vi "Measurement UI.vi"() -> ()   [LabVIEW 2021, in "Efficiency Sweep_Class D Amplifier_UI.lvlib"]
uses:
  Efficiency Sweep_Class D Amplifier_UI.lvlib
  shared/controls/units - snr.ctl
  shared/controls/units - ratio.ctl
  shared/controls/digital output level units.ctl
  shared/ui/controls/view.ctl
  shared/controls/power measurement method.ctl
  UI State.ctl
  <vilib>/Utility/miscctls.llb/LVBoundsTypeDef.ctl
  <vilib>/Utility/miscctls.llb/LVPoint32TypeDef.ctl
  <vilib>/Utility/miscctls.llb/LVPointTypeDef.ctl
  shared/ui/UI Helpers.lvlib
  shared/audio popup ui/Audio Popup UI.lvlib
  shared/controls/audio controls.lvlib
panel:
  in  "view legend":T1
  out "plot point":string
  out "Sweep graph":cluster{"frequency (Hz)":dbl[], "THD+N":dbl[]}[](graph)
  out "Time domain graph":waveform(dbl)(graph)
  out "Frequency domain graph":T2(graph)
  in  "digital serial cfg file":string
  in  "power measurement resource":string="PXI1Slot4/ai0"
  out "efficiency (%)":dbl[](array[numeric])
  out "power loss (W)":dbl[](array[numeric])
  out "total output power (W)":dbl[](array[numeric])
  out "input power (W)":dbl[](array[numeric])
  out "power supply current (A)":dbl[](array[numeric])
  out "power supply voltage (V)":dbl[](array[numeric])
  in  "Configuration tab":enum32{"Protocol", "Measurement", "Units"}(tab)
  out "digital serial file name":string
  in  "configure digital serial":bool
  in  "master clock channel list":string caption="Master Clock Channel"
  in  "digital channel list":string caption="Digital Audio Channel"
  in  "output level units 2":T3
  in  "sense resistor (Ohms)":dbl caption="Sense Resistor" format="%#_g Ohms"
  in  "power supply current limit":dbl caption="Current Limit" format="%#_g A"
  in  "power supply voltage":dbl caption="Power Supply Voltage" format="%#_g V"
  in  "power meas resource":refnum<k15> caption="Resource"
  in  "power measurement method":T4 caption="Method"
  in  "output level units":T3
  in  "min settling cycles":u32 caption="Minimum settling cycles"
  in  "min settling time (s)":dbl=0.1 caption="Minimum settling time" format="%#_6ps"
  in  "output sweep number of steps":u32=20000 caption="Number of steps"
  in  "output level start":dbl=20.0 caption="Sweep start" format="%#_6p"
  in  "output level stop":dbl=20000.0 caption="Sweep stop"
  in  "min measurement cycles":u32 caption="Minimum measurement cycles"
  in  "Acquisition channel":tag
  in  "acq sampling rate":dbl=51200.0 caption="Sample rate" format="%#.6pHz"
  in  "min measurement time (s)":dbl=0.1 caption="Minimum measurement time" format="%#_6ps"
  in  "lowpass filter":T5(ring) caption="Lowpass filter"
  in  "highpass filter":enum32{"DC", "AC"}(ring) caption="Highpass filter"
  in  "band start":dbl=20.0 caption="Band start" format="%#_6pHz"
  in  "band stop":dbl=20000.0 caption="Band stop" format="%#_6pHz"
  in  "weighting filter":T6(ring)=enum."A-weighting" caption="Weighting filter"
  in  "load impedance":dbl=4.0 caption="Load impedance" format="%#_6p Ohms"
  in  "output range (pk-pk)":dbl=15.0 caption="Output range" format="%.3p Vpk-pk"
  in  "gain units":T7 caption="Gain"
  in  "THD units":T7 caption="THD"
  in  "THD+N units":T7 caption="THD+N"
  in  "SNR units":T8 caption="SNR"
  in  "channel 0 offset":u32=1
  out "fft - data":dbl[](array[numeric])
  out "fft - df":dbl
  out "fft - f0":dbl
  out "wfm - data":dbl[](array[numeric])
  out "wfm - dt":dbl
  out "wfm - t0":dbl
  out "channel name":string
  in  "acq channel":string="PXI1Slot4/ai0"
  in  "signal phase":dbl caption="phase"
  # "hidden controls - used to sync with MeasLink"
  # "hidden indicators"
  # "Digital Serial Settings"
  # "Harware Resource"
  # "Output Sweep"
  # "Filters"
  # "Acquisition"
  # "Power"
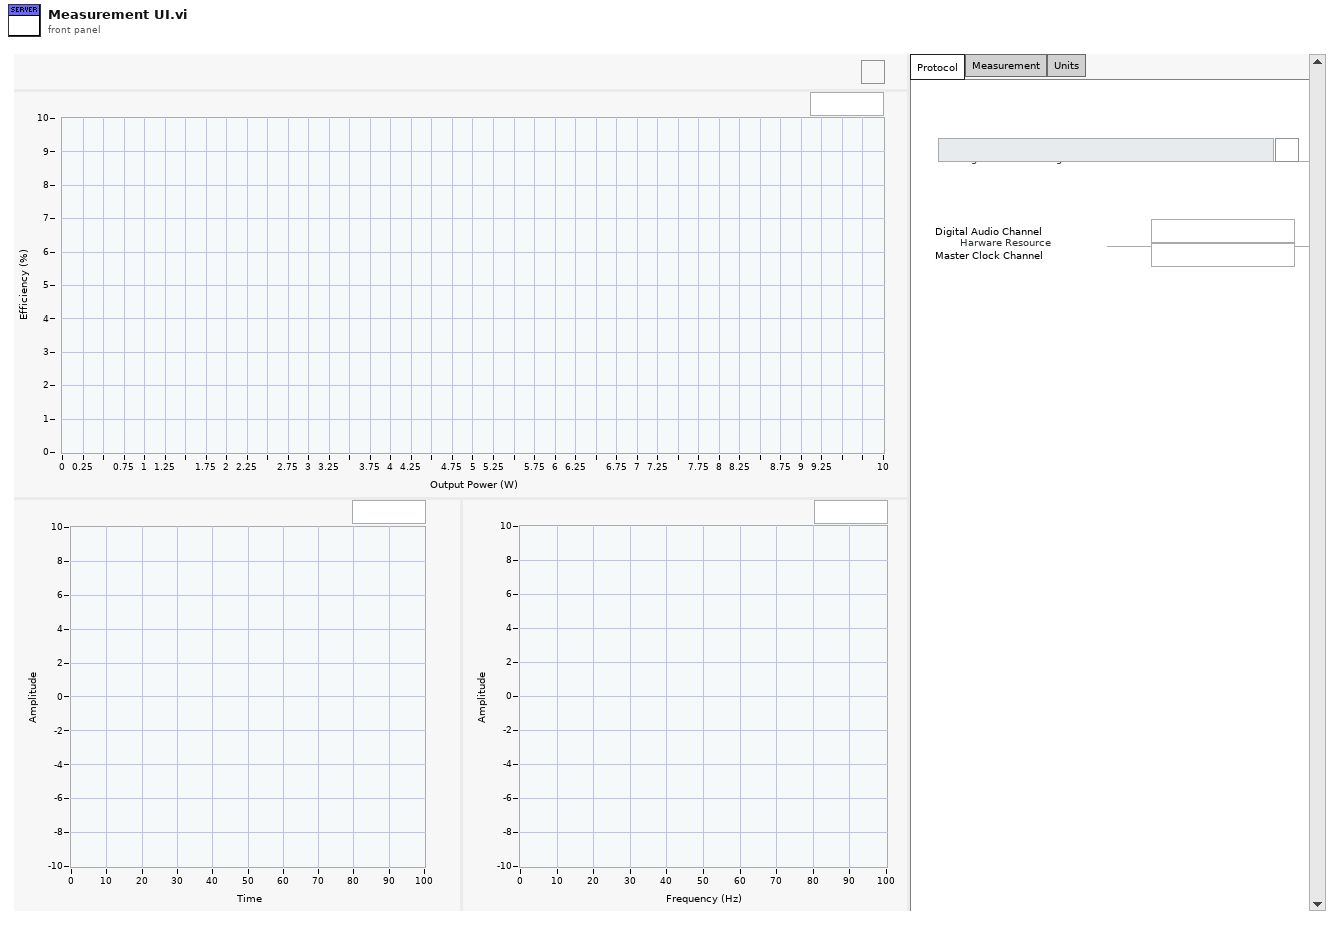
[diagram p1: front panel]
types:
  T1 = typedef "UI Helpers.lvlib/view.ctl" = bool
  T2 = cluster{"fft - f0":dbl, "fft - df":dbl, "fft - data":dbl[]}
  T3 = typedef "audio controls.lvlib/digital output level units.ctl" = enum32{"% FS", "dBFS", "V"}
  T4 = typedef "power measurement method.ctl" = enum32{"SMU", "DMM"}
  T5 = enum32{"No filter", "AES17 20kHz", "AES17 40kHz"}
  T6 = enum32{"Linear", "A-weighting", "B-weighting", "C-weighting"}
  T7 = typedef "audio controls.lvlib/units - ratio.ctl" = enum32{"dB", "%", "x/y"}
  T8 = typedef "audio controls.lvlib/units - snr.ctl" = enum32{"dB", "x/y"}
  T9 = typedef "Efficiency Sweep_Class D Amplifier_UI.lvlib/UI State.ctl" = cluster{"Graph Size":T10, "Legend Visible":bool, "Mouse Coords":T11, "Visible Plot Id":i32, "PostUI event occurred":bool, "digital serial cfg file":path}
  T10 = typedef "LVBoundsTypeDef.ctl" = cluster{"Width":u32, "Height":u32}
  T11 = typedef "LVPoint32TypeDef.ctl" = cluster{"Horizontal":i32, "Vertical":i32}
  T12 = typedef "LVPointTypeDef.ctl" = cluster{"Horizontal":i16, "Vertical":i16}
  T13 = typedef "Audio Popup UI.lvlib/audio settings.ctl" = cluster{"digital serial file":string}
  T14 = cluster{"total output power (W)":dbl[], "efficiency (%)":dbl[]}
  T15 = cluster{"total output power (W)":dbl[], "power loss (W)":dbl[]}
  T16 = cluster{"total output power (W)":dbl[], "input power (W)":dbl[]}
  T17 = cluster{"total output power (W)":dbl[], "input power (W)":dbl[]}[]
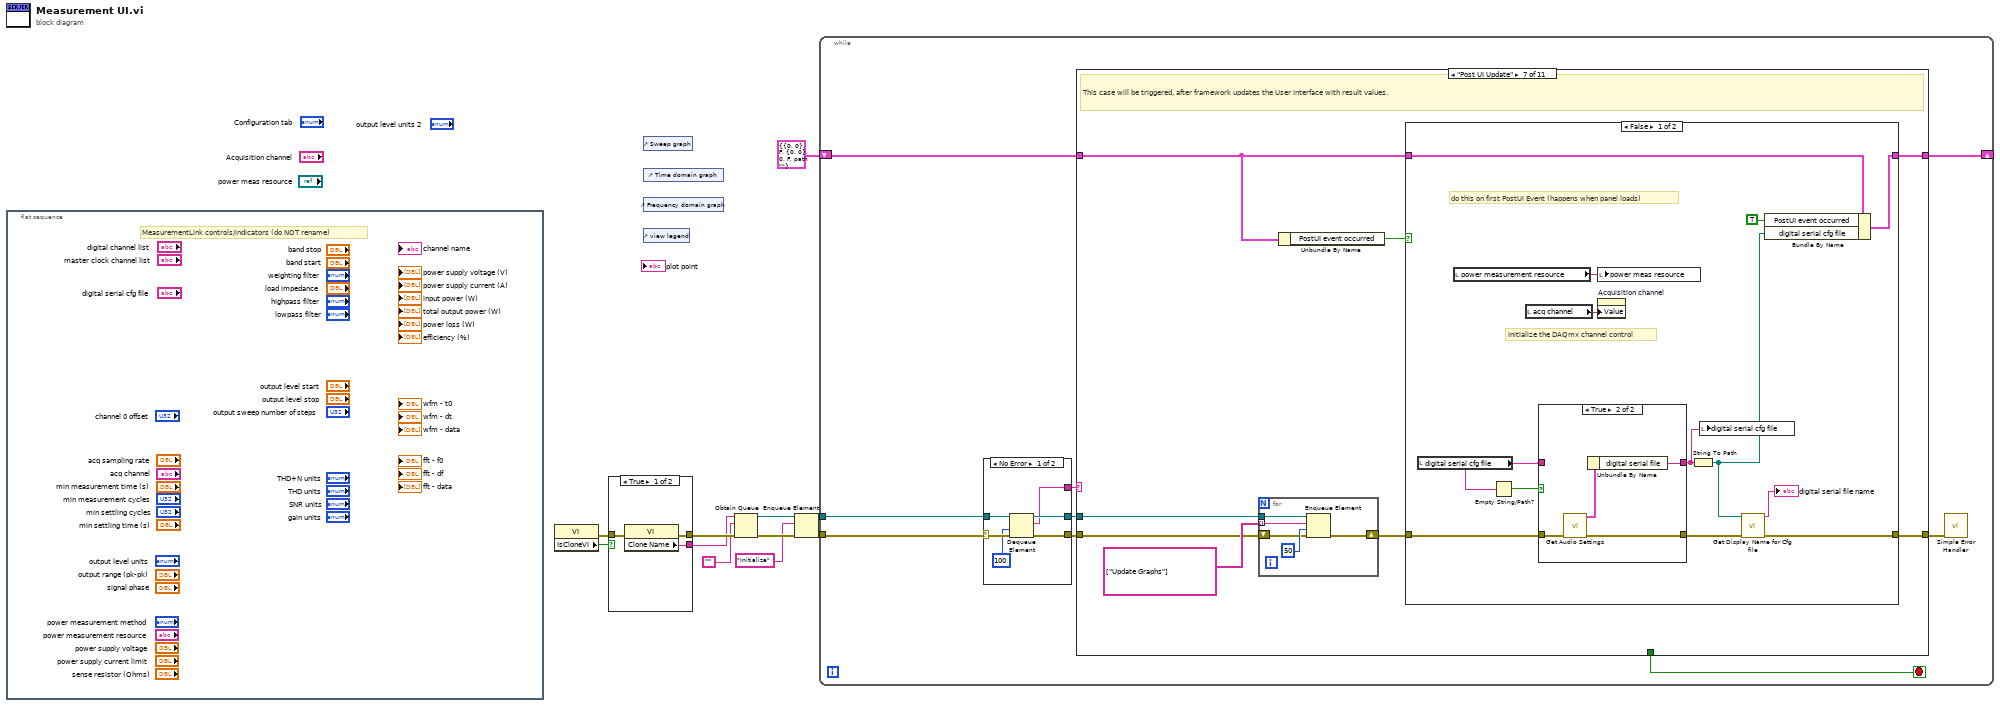
[diagram p0: block diagram]
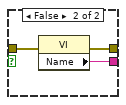
[diagram p2: hidden frame]
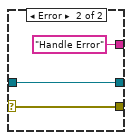
[diagram p3: hidden frame]
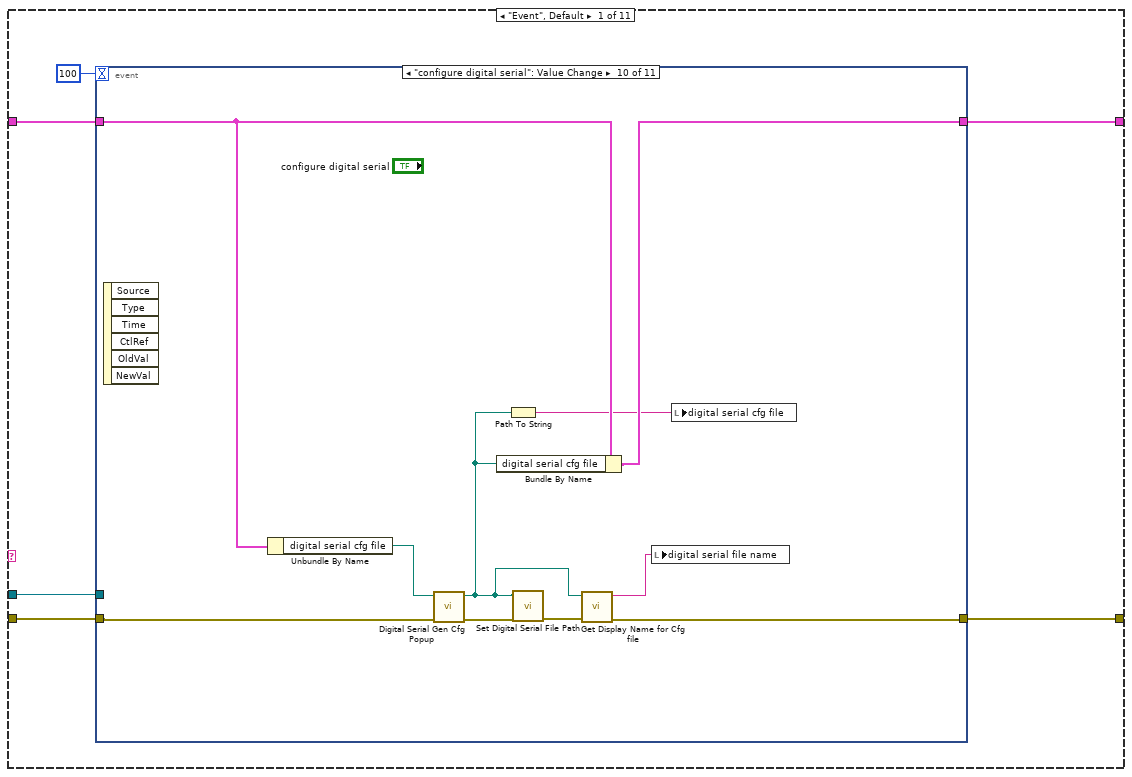
[diagram p4: hidden frame]
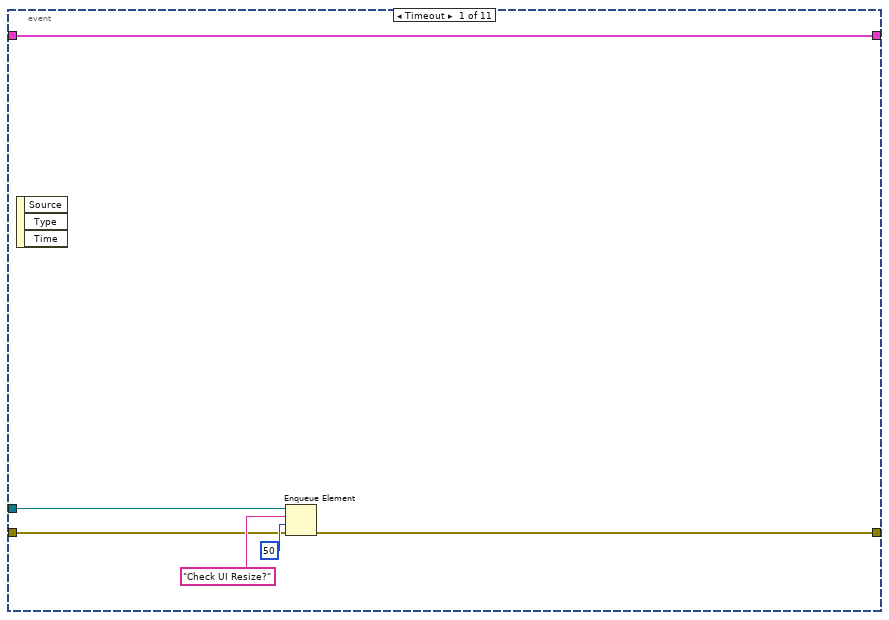
[diagram p5: hidden frame]
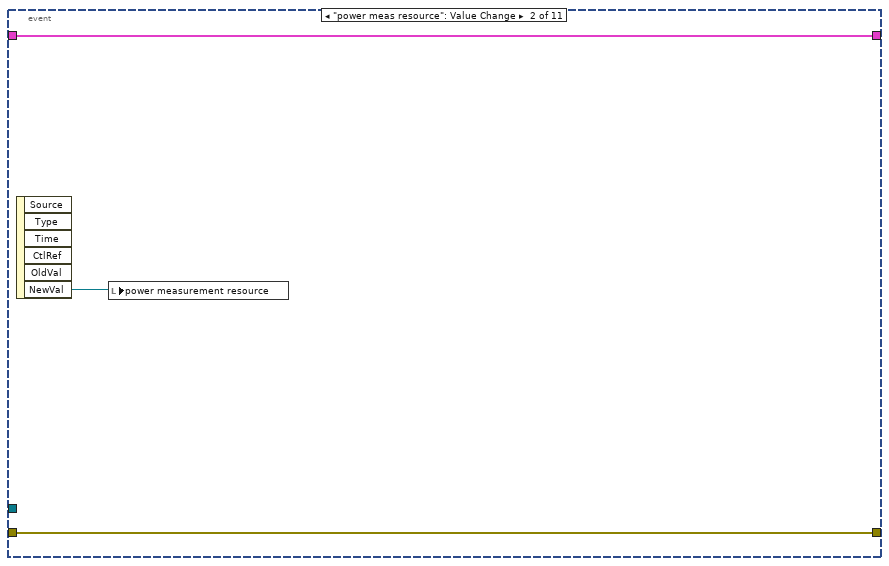
[diagram p6: hidden frame]
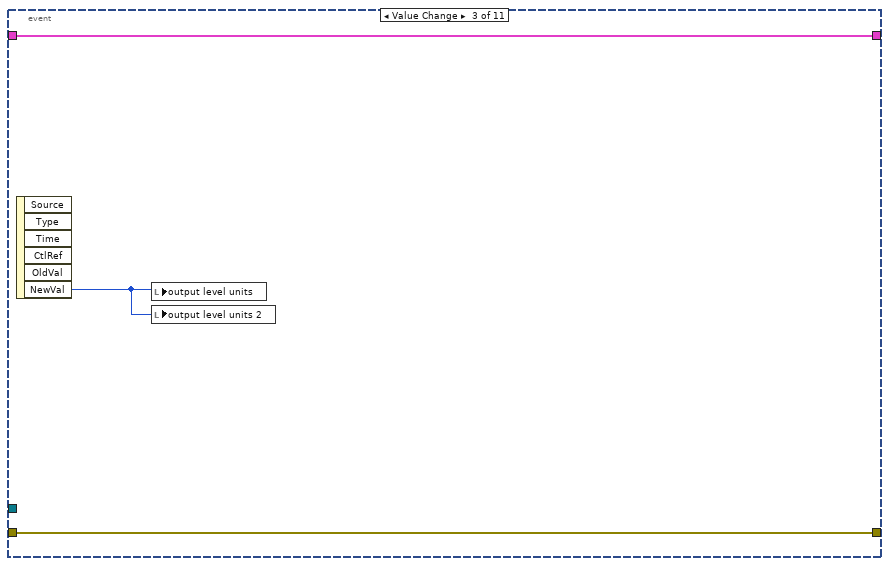
[diagram p7: hidden frame]
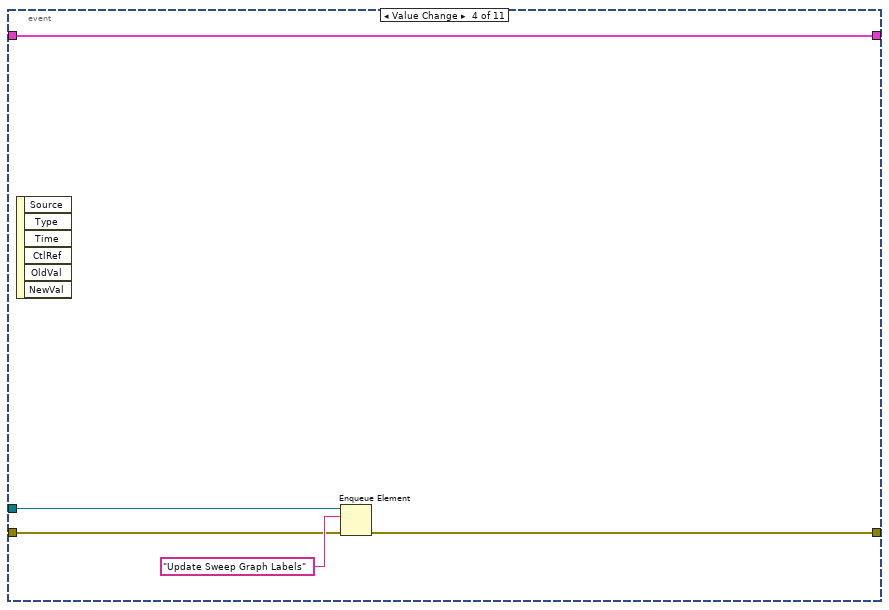
[diagram p8: hidden frame]
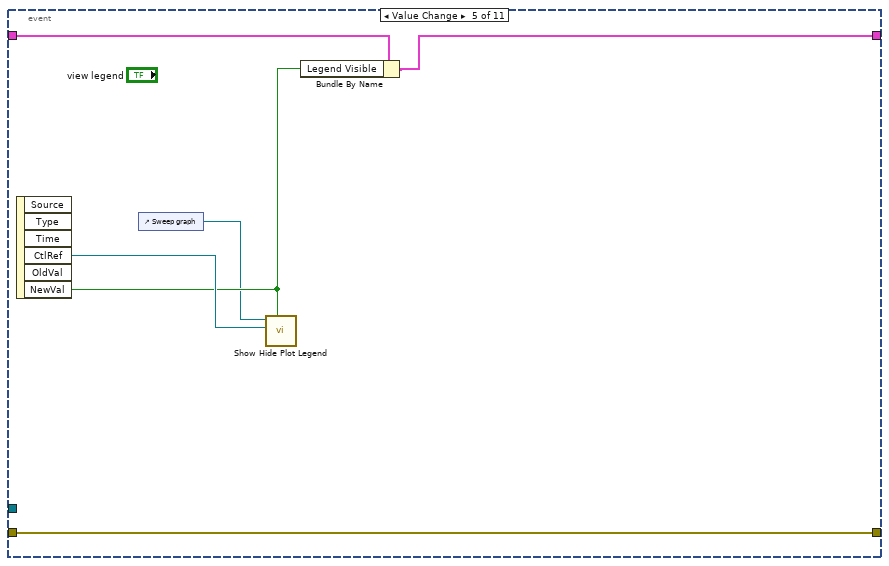
[diagram p9: hidden frame]
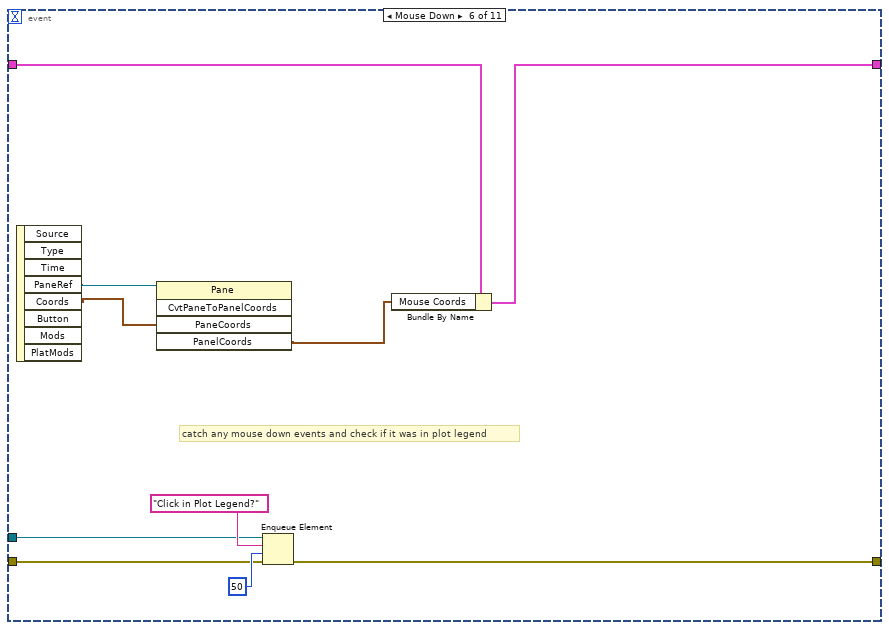
[diagram p10: hidden frame]
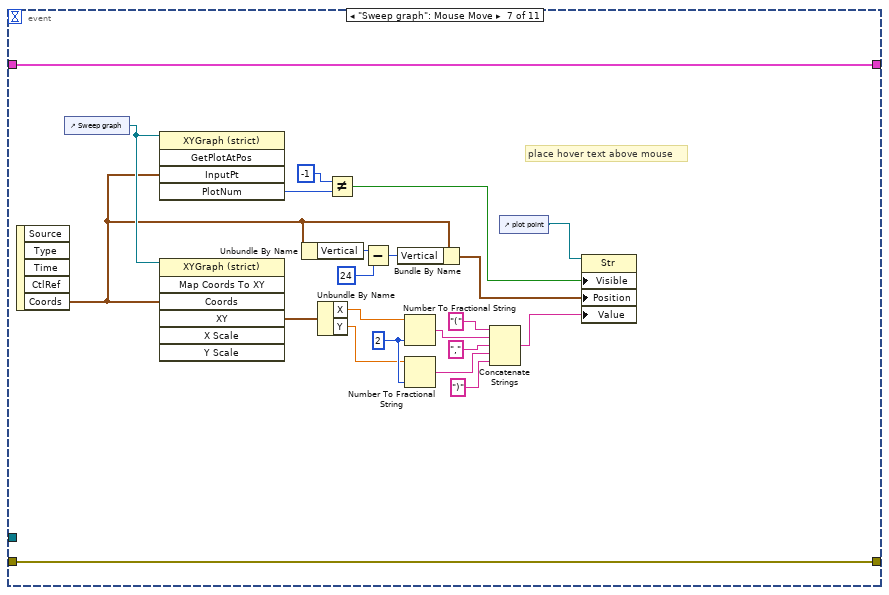
[diagram p11: hidden frame]
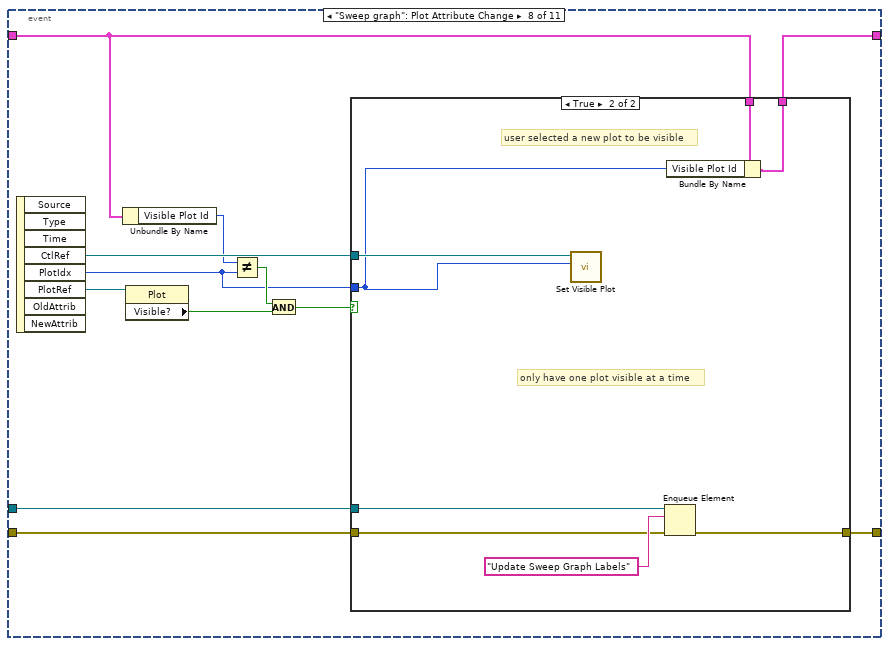
[diagram p12: hidden frame]
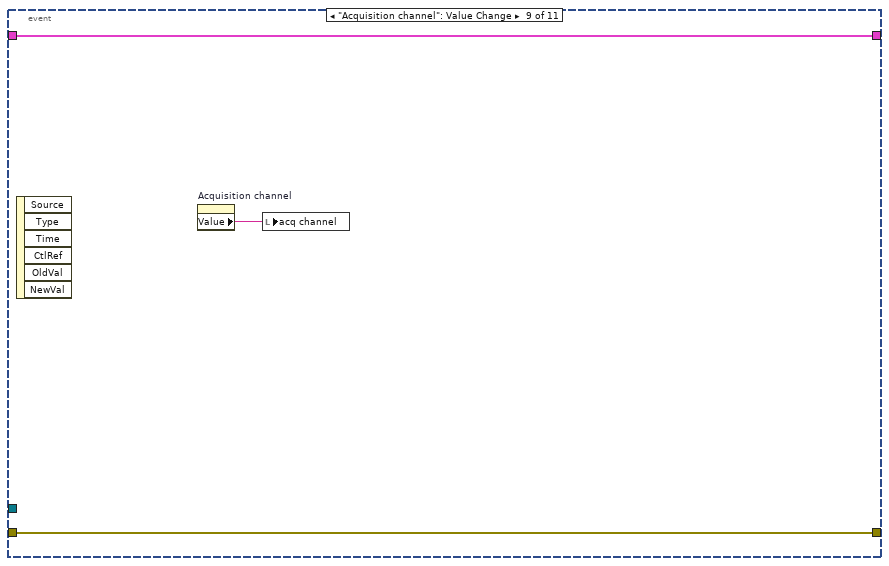
[diagram p14: hidden frame]
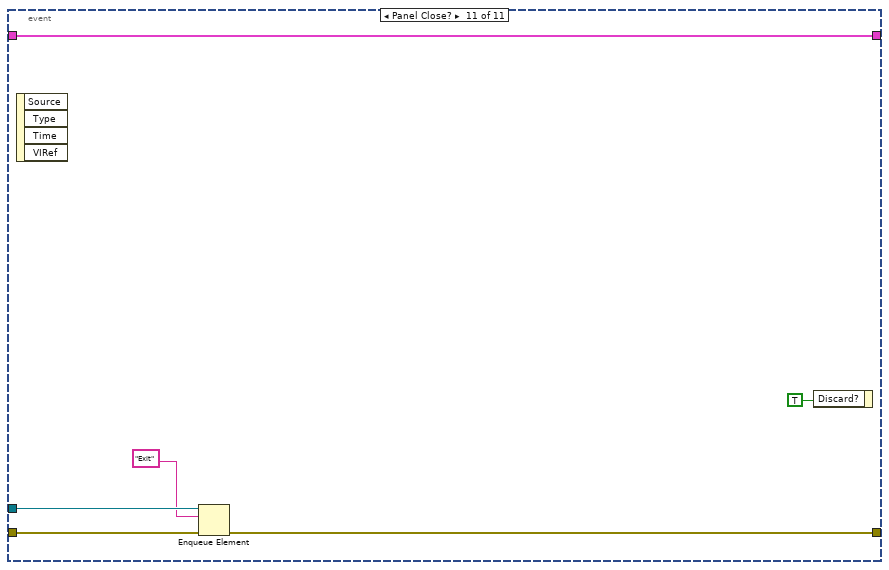
[diagram p15: hidden frame]
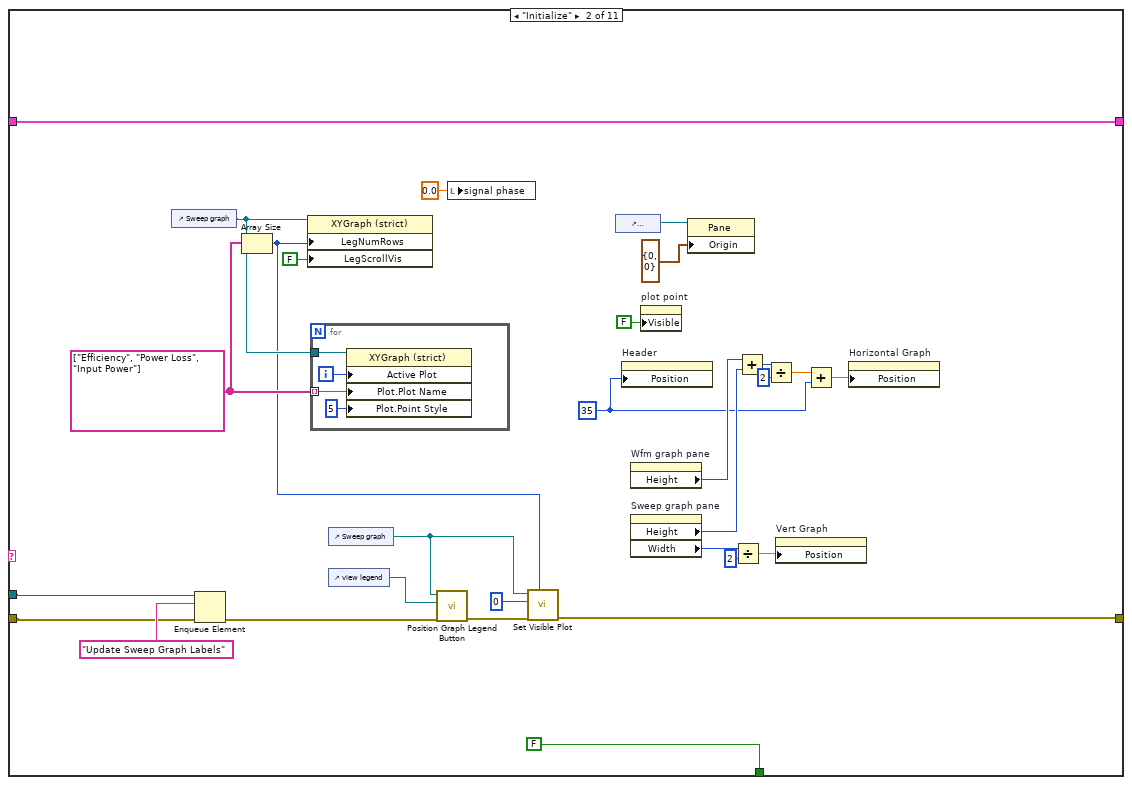
[diagram p16: hidden frame]
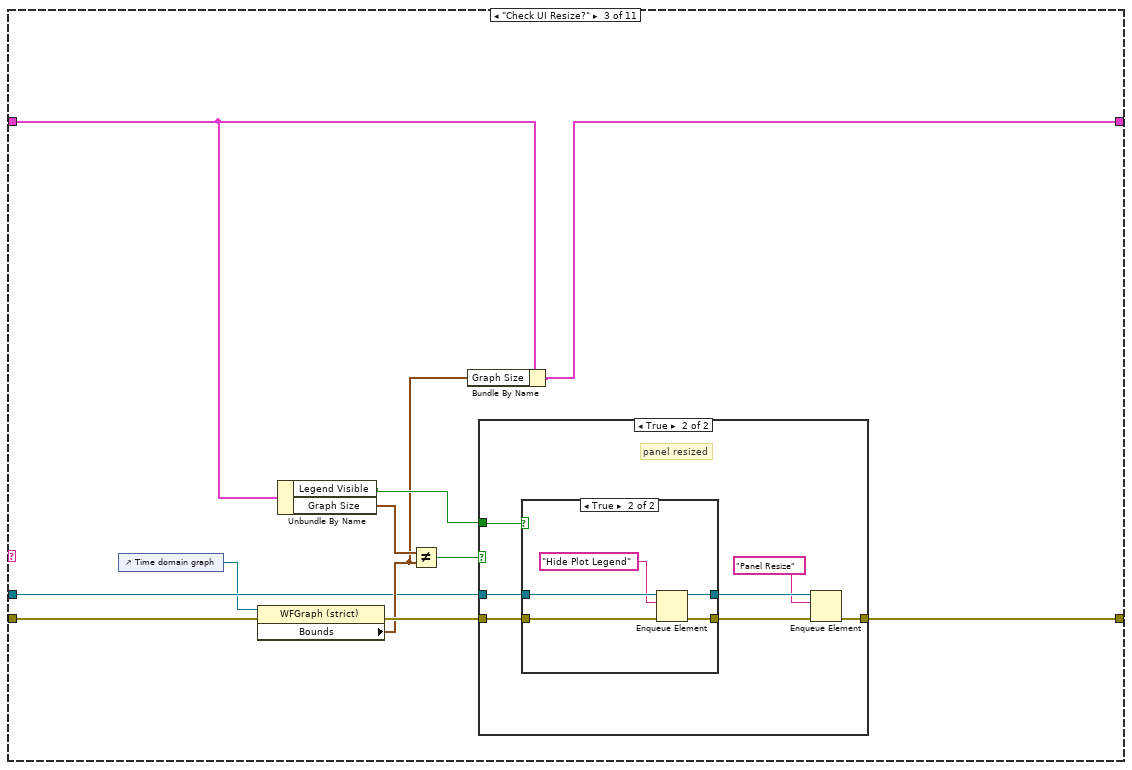
[diagram p17: hidden frame]
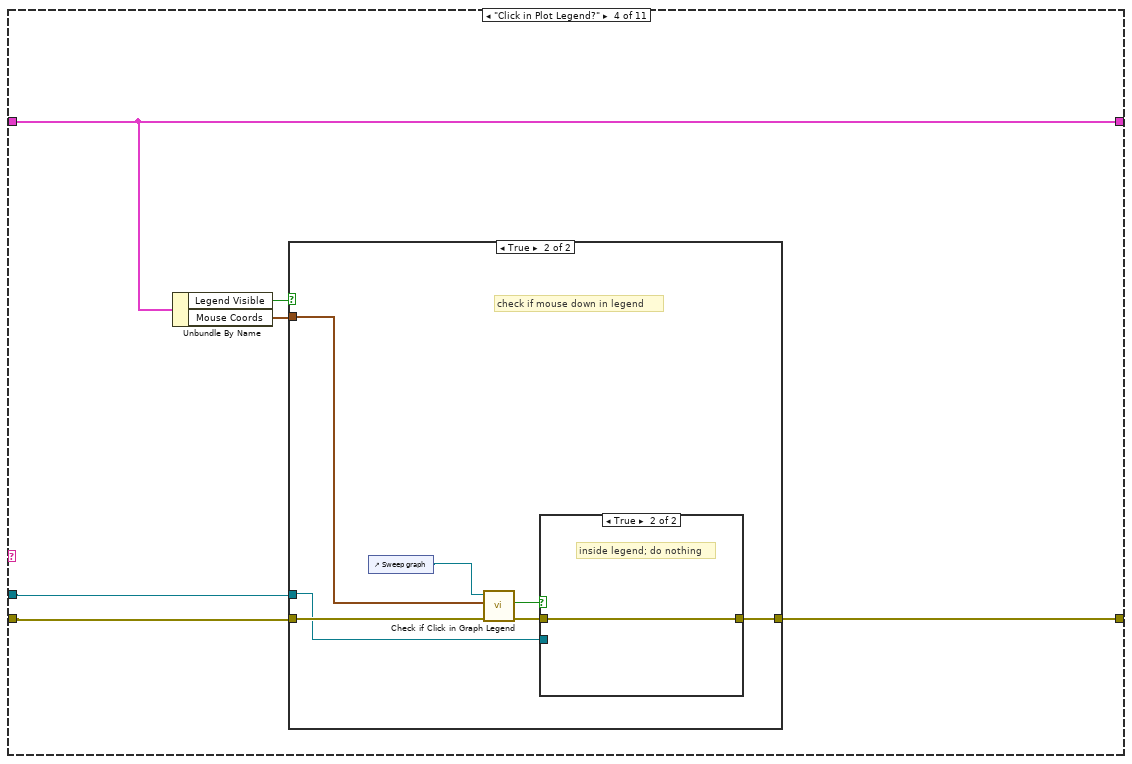
[diagram p20: hidden frame]
diagram:
  n1 = flat-sequence {
    frame #0 {
      # "MeasurementLink controls/indicators (do NOT rename)"
    }
  }
  n2 = property class="VI"() -> (error out=w2:errorcluster, "IsCloneVI"=w3:bool)  [unwired: 2 in, 1 out]
  n3 = case shown="True" w3 {
    tunnel: [w14 w17] -> w11
    tunnel: [w13 w16] -> w10
    tunnel: w2 -> [w12 w15]
    frame True {
      n4 = property class="VI"(error in=w12) -> (error out=w14:errorcluster, "Clone Name"=w13:string)  [unwired: 1 in, 1 out]
    }
    frame False {
      n5 = property class="VI"(error in=w15) -> (error out=w17:errorcluster, "Name"=w16:string)  [unwired: 1 in, 1 out]
    }
  }
  n6 = control-ref of="Sweep graph"() -> ()  [unwired: 1 out]
  n7 = control-ref of="Time domain graph"() -> ()  [unwired: 1 out]
  n8 = control-ref of="Frequency domain graph"() -> ()  [unwired: 1 out]
  n9 = control-ref of="view legend"() -> ()  [unwired: 1 out]
  n10 = Obtain Queue(name (unnamed)=w10, element data type="", error in (no error)=w11) -> (queue out=w7:refnum<queue>, error out=w9:errorcluster)  [unwired: 2 in, 1 out]
  n11 = Enqueue Element(queue=w7, element="Initialize", error in (no error)=w9) -> (queue out=w6:refnum<queue>, error out=w8:errorcluster)  [unwired: 1 in, 1 out]
  n12 = while {
    tunnel: w6 -> [w24]
    shift-right: [w20] -> _
    shift-left: T9 {"Graph Size"={"Width"=0, "Height"=0}, "Legend Visible"=FALSE, "Mouse Coords"={"Horizontal"=0, "Vertical"=0}, "Visible Plot Id"=0, "PostUI event occurred"=FALSE, "digital serial cfg file"=path ""} ("UI State") -> [w19]
    tunnel: w8 -> [w26]
    stop <- w21 stop-if-true
    n13 = case shown="No Error" w26 {
      selector: w26 -> [w32 w35]
      tunnel: [w31 w35] -> w25
      tunnel: w24 -> [w30 w34]
      tunnel: [w29 w34] -> w23
      tunnel: [w28 "Handle Error"] -> w22
      frame No Error {
        n14 = Dequeue Element(queue=w30, timeout in ms (-1)=100, error in (no error)=w32) -> (queue out=w29:refnum<queue>, element=w28:string, error out=w31:errorcluster)  [unwired: 1 out]
      }
      frame Error {
      }
    }
    n15 = case shown="\"Post UI Update\"" w22 {
      tunnel: w25 -> [w40 w146 w175 w199 w219 w227 w235 w272 w284 w292 w294]
      tunnel: w23 -> [w38 w147 w176 w200 _ _ w234 _ _ w290 _]
      tunnel: [w41 w153 w174 w198 w218 w226 w229 w272 w284 w287 w294] -> w18
      tunnel: [_ FALSE _ _ _ _ _ _ _ TRUE _] -> w21
      tunnel: [w36 w138 w171 w197 w221 w228 w232 w271 w283 w285 w293] -> w20
      tunnel: w19 -> [w37 w138 w172 w197 w222 w228 w233 w271 w283 w285 w293]
      frame "Event", Default {
        n16 = event shown="[9] \"configure digital serial\": Value Change" {
          selector: _ -> [_ _ _ _ _ _ _ _ _ _ _]
          dyn-events: _ -> [_ _ _ _ _ _ _ _ _ _ _]
          timeout: 100 -> [_ _ _ _ _ _ _ _ _ _ _]
          tunnel: [w44 w50 w53 w54 w64 w70 w96 w104 w119 w122 w135] -> w41
          tunnel: w40 -> [w45 w50 w53 w55 w64 w72 w96 w106 w119 w127 w136]
          tunnel: w38 -> [w43 _ _ w56 _ w71 _ w105 _ _ w134]
          tunnel: w37 -> [w42 w49 w52 w58 w61 w69 w95 w99 w120 w126 w132]
          tunnel: [w42 w49 w52 w58 w60 w68 w95 w98 w120 w125 w132] -> w36
          event Timeout {
            n17 = event-data() -> ()  [unwired: 1 in, 3 out]
            n18 = Enqueue Element(queue=w43, element="Check UI Resize?", timeout in ms (-1)=50, error in (no error)=w45) -> (error out=w44:errorcluster)  [unwired: 2 out]
          }
          event "power meas resource": Value Change {
            n19 = event-data() -> ("NewVal"=w48:refnum<k15>)  [unwired: 1 in, 5 out]
            n20 = local write "power measurement resource"(w48) -> ()
          }
          event Value Change {
            n21 = event-data() -> ("NewVal"=w51:T3)  [unwired: 1 in, 5 out]
            n22 = local write "output level units"(w51) -> ()
            n23 = local write "output level units 2"(w51) -> ()
          }
          event Value Change {
            n24 = event-data() -> ()  [unwired: 1 in, 6 out]
            n25 = Enqueue Element(queue=w56, element="Update Sweep Graph Labels", error in (no error)=w55) -> (error out=w54:errorcluster)  [unwired: 1 in, 2 out]
          }
          event Value Change {
            n26 = event-data() -> ("CtlRef"=w63:refnum<vi>, "NewVal"=w62:T1)  [unwired: 1 in, 4 out]
            n27 = control-ref of="Sweep graph"() -> (w59:refnum<vi>)
            n28 = call "Show Hide Plot Legend.vi"("show"=w62, "view reference"=w63, "graph reference"=w59) -> ()  [unwired: 8 in, 1 out]
            n29 = Bundle By Name(cluster=w61, "Legend Visible"=w62) -> (w60:T9)
          }
          event Mouse Down {
            # "catch any mouse down events and check if it was in plot legend"
            n30 = event-data() -> ("PaneRef"=w67:refnum<vi>, "Coords"=w66:T11)  [unwired: 1 in, 6 out]
            n31 = invoke class="Pane" method="CvtPaneToPanelCoords"(reference=w67, "PaneCoords"=w66) -> ("PanelCoords"=w65:T12)  [unwired: 3 in, 4 out]
            n32 = Enqueue Element(queue=w71, element="Click in Plot Legend?", timeout in ms (-1)=50, error in (no error)=w72) -> (error out=w70:errorcluster)  [unwired: 2 out]
            n33 = Bundle By Name(cluster=w69, "Mouse Coords"=w65) -> (w68:T9)
          }
          event "Sweep graph": Mouse Move {
            w85 = i16 2 ("precision (6)")
            # "place hover text above mouse"
            n34 = event-data() -> ("Coords"=w75:T11)  [unwired: 1 in, 4 out]
            n35 = control-ref of="Sweep graph"() -> (w76:refnum<vi>)
            n36 = invoke class="XYGraph (strict)" method="GetPlotAtPos"(reference=w76, "InputPt"=w75) -> ("PlotNum"=w93:i32)  [unwired: 3 in, 4 out]
            n37 = invoke class="XYGraph (strict)" method="Map Coords To XY"(reference=w76, "Coords"=w75) -> ("XY"=w94:cluster{"X":dbl, "Y":dbl})  [unwired: 5 in, 6 out]
            n38 = Unbundle By Name(w75) -> ("Vertical"=w80:i32)
            n39 = Unbundle By Name(w94) -> ("X"=w83:dbl, "Y"=w82:dbl)
            n40 = Not Equal?(x=-1, y=w93) -> (x != y?=w91:bool)
            n41 = Subtract(x=w80, y=24) -> (x-y=w79:i32)
            n42 = Bundle By Name(cluster=w75, "Vertical"=w79) -> (w81:T11)
            n43 = Number To Fractional String(number=w83, precision (6)=w85) -> (F-format string=w89:string)  [unwired: 2 in]
            n44 = Number To Fractional String(number=w82, precision (6)=w85) -> (F-format string=w87:string)  [unwired: 2 in]
            n45 = Concatenate Strings("(" ("string"), w89, "," ("string"), w87, ")" ("string")) -> (w84:string)
            n46 = control-ref of="plot point"() -> (w77:refnum<vi>)
            n47 = property on="Property Node" class="Str"(reference=w77, "Visible"=w91, "Position"=w81, "Value"=w84) -> ()  [unwired: 1 in, 2 out]
          }
          event "Sweep graph": Plot Attribute Change {
            n48 = event-data() -> ("CtlRef"=w107:refnum<vi>, "PlotIdx"=w97:i32, "PlotRef"=w108:refnum<vi>)  [unwired: 1 in, 5 out]
            n49 = Unbundle By Name(w99) -> ("Visible Plot Id"=w103:i32)
            n50 = property class="Plot"(reference=w108) -> ("Visible?"=w101:bool)  [unwired: 1 in, 2 out]
            n51 = Not Equal?(x=w103, y=w97) -> (x != y?=w102:bool)
            n52 = And(x=w102, y=w101) -> (x .and. y?=w100:bool)
            n53 = case shown="True" w100 {
              tunnel: w107 -> [_ w118]
              tunnel: w106 -> [w110 w116]
              tunnel: w105 -> [_ w115]
              tunnel: [w110 w114] -> w104
              tunnel: w99 -> [w109 w113]
              tunnel: [w109 w112] -> w98
              tunnel: w97 -> [_ w111]
              frame False {
              }
              frame True {
                # "only have one plot visible at a time"
                # "user selected a new plot to be visible"
                n54 = call "Set Visible Plot.vi"("Plot Id"=w111, "XYGraph in"=w118) -> ()  [unwired: 9 in, 1 out]
                n55 = Enqueue Element(queue=w115, element="Update Sweep Graph Labels", error in (no error)=w116) -> (error out=w114:errorcluster)  [unwired: 1 in, 2 out]
                n56 = Bundle By Name(cluster=w113, "Visible Plot Id"=w111) -> (w112:T9)
              }
            }
          }
          event "Acquisition channel": Value Change {
            n57 = event-data() -> ()  [unwired: 1 in, 6 out]
            n58 = property on="Acquisition channel" class="DAQmxName"() -> ("Value"=w121:string)  [unwired: 2 in, 2 out]
            n59 = local write "acq channel"(w121) -> ()
          }
          event "configure digital serial": Value Change {
            n60 = event-data() -> ()  [unwired: 1 in, 6 out]
            n61 = Unbundle By Name(w126) -> ("digital serial cfg file"=w131:path)
            n62 = call "Digital Serial Gen Cfg Popup.vi"("error in (no error)"=w127, "config file in"=w131) -> ("error out"=w130:errorcluster, "config file out"=w128:path)  [unwired: 7 in, 1 out]
            n63 = Bundle By Name(cluster=w126, "digital serial cfg file"=w128) -> (w125:T9)
            n64 = Path To String(path=w128) -> (string=w124:string)
            n65 = call "Set Digital Serial File Path.vi"("error in (no error)"=w130, "digital serial file"=w128) -> ("error out"=w129:errorcluster)  [unwired: 9 in]
            n66 = call "Get Display Name for Cfg file.vi"("error in (no error)"=w129, "file path"=w128) -> ("error out"=w122:errorcluster, "display string"=w123:string)  [unwired: 8 in]
            n67 = local write "digital serial file name"(w123) -> ()
            n68 = local write "digital serial cfg file"(w124) -> ()
          }
          event Panel Close? {
            n69 = event-data() -> ()  [unwired: 1 in, 4 out]
            n70 = Enqueue Element(queue=w134, element="Exit", error in (no error)=w136) -> (error out=w135:errorcluster)  [unwired: 1 in, 2 out]
            n71 = event-data("Discard?"=TRUE) -> ()  [unwired: 1 in, 1 out]
          }
        }
      }
      frame "Initialize" {
        w144 = 35 ("Splitter Position")
        w141 = string[] ["Efficiency", "Power Loss", "Input Power"]
        n72 = control-ref of="Sweep graph"() -> (w150:refnum<vi>)
        n73 = Enqueue Element(queue=w147, element="Update Sweep Graph Labels", error in (no error)=w146) -> (error out=w145:errorcluster)  [unwired: 1 in, 2 out]
        n74 = Array Size(array=w141) -> (size(s)=w140:i32)
        n75 = property class="XYGraph (strict)"(reference=w150, "LegNumRows"=w140, "LegScrollVis"=FALSE ("Legend:Scrollbar Visible")) -> ()  [unwired: 1 in, 2 out]
        n76 = for {
          tunnel: w141 -> [w169] mode=indexing
          tunnel: w150 -> [w168]
          i -> [w170]
          n77 = property on="Property Node" class="XYGraph (strict)"(reference=w168, "Active Plot"=w170, "Plot.Plot Name"=w169, "Plot.Point Style"=u8 5) -> ()  [unwired: 1 in, 2 out]
        }
        n78 = control-ref of="Sweep graph"() -> (w152:refnum<vi>)
        n79 = control-ref of="view legend"() -> (w164:refnum<vi>)
        n80 = call "Position Graph Legend Button.vi"("error in (no error)"=w145, "view legend"=w164, "graph"=w152) -> ("error out"=w154:errorcluster)  [unwired: 8 in]
        n81 = local write "signal phase"(0.0 ("signal phase")) -> ()
        n82 = call "Set Visible Plot.vi"("number of plots"=w140, "error in (no error)"=w154, "Plot Id"=0, "XYGraph in"=w152) -> ("error out"=w153:errorcluster)  [unwired: 7 in]
        n83 = control-ref of="Configuration Pane"() -> (w143:refnum<vi>)
        n84 = property on="Header" class="Splitter"("Position"=w144) -> ()  [unwired: 2 in, 2 out]
        n85 = property on="Wfm graph pane" class="Pane"() -> ("Height"=w157:u32)  [unwired: 2 in, 2 out]
        n86 = property on="Sweep graph pane" class="Pane"() -> ("Height"=w156:u32, "Width"=w159:u32)  [unwired: 2 in, 2 out]
        n87 = property on="plot point" class="Str"("Visible"=FALSE) -> ()  [unwired: 2 in, 2 out]
        n88 = property class="Pane"(reference=w143, "Origin"=T12 {"Horizontal"=0, "Vertical"=0}) -> ()  [unwired: 1 in, 2 out]
        n89 = Divide(x=w159, y=2) -> (x/y=w158:dbl)
        n90 = Add(x=w157, y=w156) -> (x+y=w155:u32)
        n91 = Divide(x=w155, y=2) -> (x/y=w162:dbl)
        n92 = property on="Vert Graph" class="Splitter"("Position"=w158) -> ()  [unwired: 2 in, 2 out]
        n93 = Add(x=w162, y=w144) -> (x+y=w161:dbl)
        n94 = property on="Horizontal Graph" class="Splitter"("Position"=w161) -> ()  [unwired: 2 in, 2 out]
      }
      frame "Check UI Resize?" {
        n95 = control-ref of="Time domain graph"() -> (w173:refnum<vi>)
        n96 = property on="Property Node" class="WFGraph (strict)"(reference=w173, error in=w175) -> (error out=w181:errorcluster, "Bounds"=w177:T10)  [unwired: 1 out]
        n97 = Unbundle By Name(w172) -> ("Legend Visible"=w179:bool, "Graph Size"=w178:T10)
        n98 = Not Equal?(x=w178, y=w177) -> (x != y?=w180:bool)
        n99 = Bundle By Name(cluster=w172, "Graph Size"=w177) -> (w171:T9)
        n100 = case shown="True" w180 {
          tunnel: w181 -> [w182 w189]
          tunnel: [w182 w184] -> w174
          tunnel: w179 -> [_ w187]
          tunnel: w176 -> [_ w188]
          frame False {
            # "no resize"
          }
          frame True {
            # "panel resized"
            n101 = case shown="True" w187 {
              tunnel: w189 -> [w191 w196]
              tunnel: [w191 w195] -> w186
              tunnel: w188 -> [w190 w194]
              tunnel: [w190 w192] -> w185
              frame False {
              }
              frame True {
                n102 = Enqueue Element(queue=w194, element="Hide Plot Legend", error in (no error)=w196) -> (queue out=w192:refnum<queue>, error out=w195:errorcluster)  [unwired: 1 in, 1 out]
              }
            }
            n103 = Enqueue Element(queue=w185, element="Panel Resize", error in (no error)=w186) -> (error out=w184:errorcluster)  [unwired: 1 in, 2 out]
          }
        }
      }
      frame "Click in Plot Legend?" {
        n104 = Unbundle By Name(w197) -> ("Legend Visible"=w201:bool, "Mouse Coords"=w202:T11)
        n105 = case shown="True" w201 {
          tunnel: w202 -> [_ w209]
          tunnel: w200 -> [_ w206]
          tunnel: w199 -> [w203 w210]
          tunnel: [w203 w205] -> w198
          frame False {
            # "legend not visible; do nothing"
          }
          frame True {
            # "check if mouse down in legend"
            n106 = control-ref of="Sweep graph"() -> (w204:refnum<vi>)
            n107 = call "Check if Click in Graph Legend.vi"("error in (no error)"=w210, "Mouse Coords"=w209, "WaveformGraph"=w204) -> ("error out"=w207:errorcluster, "click in legend?"=w208:bool)  [unwired: 7 in]
            n108 = case shown="True" w208 {
              tunnel: w207 -> [w214 w215]
              tunnel: w206 -> [w213 _]
              tunnel: [w212 w215] -> w205
              frame False {
                n109 = Enqueue Element(queue=w213, element="Hide Plot Legend", error in (no error)=w214) -> (error out=w212:errorcluster)  [unwired: 1 in, 2 out]
              }
              frame True {
                # "inside legend; do nothing"
              }
            }
          }
        }
      }
      frame "Hide Plot Legend" {
        n110 = control-ref of="Sweep graph"() -> (w216:refnum<vi>)
        n111 = control-ref of="view legend"() -> (w217:refnum<vi>)
        n112 = call "Show Hide Plot Legend.vi"("show"=FALSE, "error in (no error)"=w219, "view reference"=w217, "graph reference"=w216) -> ("error out"=w218:errorcluster)  [unwired: 7 in]
        n113 = Bundle By Name(cluster=w222, "Legend Visible"=FALSE ("legend visible")) -> (w221:T9)
      }
      frame "Panel Resize" {
        n114 = control-ref of="Sweep graph"() -> (w225:refnum<vi>)
        n115 = control-ref of="view legend"() -> (w224:refnum<vi>)
        n116 = call "Position Graph Legend Button.vi"("error in (no error)"=w227, "view legend"=w224, "graph"=w225) -> ("error out"=w226:errorcluster)  [unwired: 8 in]
      }
      frame "Post UI Update" {
        # "This case will be triggered, after framework updates the User interface with result values."
        n117 = for {
          tunnel: w234 -> [w260]
          shift-right: [w259] -> w230
          shift-left: w235 -> [w261]
          tunnel: string[] ["Update Graphs"] -> [w258] mode=indexing
          n118 = Enqueue Element(queue=w260, element=w258, timeout in ms (-1)=50, error in (no error)=w261) -> (error out=w259:errorcluster)  [unwired: 2 out]
        }
        n119 = Unbundle By Name(w233) -> ("PostUI event occurred"=w231:bool)
        n120 = case shown="False" w231 {
          tunnel: w233 -> [w249 w257]
          tunnel: [w248 w257] -> w232
          tunnel: w230 -> [w243 w256]
          tunnel: [w238 w256] -> w229
          frame False {
            # "Initialize the DAQmx channel control"
            # "do this on first PostUI Event (happens when panel loads)"
            n121 = local read "digital serial cfg file"() -> (w240:string)
            n122 = local read "power measurement resource"() -> (w246:string)
            n123 = Empty String/Path?(string/path=w240) -> (empty?=w239:bool)
            n124 = local read "acq channel"() -> (w245:string)
            n125 = case shown="True" w239 {
              tunnel: w243 -> [w251 w255]
              tunnel: [w251 w253] -> w244
              tunnel: w240 -> [w250 _]
              tunnel: [w250 w252] -> w241
              frame False {
              }
              frame True {
                n126 = call "Get Audio Settings.vi"("error in (no error)"=w255) -> ("error out"=w253:errorcluster, "audio settings"=w254:T13)  [unwired: 9 in]
                n127 = Unbundle By Name(w254) -> ("digital serial file"=w252:string)
              }
            }
            n128 = local write "power meas resource"(w246) -> ()
            n129 = property on="Acquisition channel" class="DAQmxName"("Value"=w245) -> ()  [unwired: 2 in, 2 out]
            n130 = String To Path(string=w241) -> (path=w242:path)
            n131 = local write "digital serial cfg file"(w241) -> ()
            n132 = call "Get Display Name for Cfg file.vi"("error in (no error)"=w244, "file path"=w242) -> ("error out"=w238:errorcluster, "display string"=→"digital serial file name":string)  [unwired: 8 in]
            n133 = Bundle By Name(cluster=w249, "PostUI event occurred"=TRUE, "digital serial cfg file"=w242) -> (w248:T9)
          }
          frame True {
          }
        }
      }
      frame "Update Graphs" {
        n134 = disable-structure shown="Disabled" {
          frame Disabled {
            # "maybe use for debugging ???"
            n135 = local read "power supply voltage (V)"() -> ()  [unwired: 1 out]
            n136 = local read "power supply current (A)"() -> ()  [unwired: 1 out]
          }
          frame Enabled {
          }
        }
        n137 = local read "total output power (W)"() -> (w266:dbl[])
        n138 = local read "input power (W)"() -> (w263:dbl[])
        n139 = local read "power loss (W)"() -> (w264:dbl[])
        n140 = local read "efficiency (%)"() -> (w265:dbl[])
        n141 = local read "wfm - data"() -> (w278:dbl[])
        n142 = local read "fft - data"() -> (w275:dbl[])
        n143 = local read "wfm - dt"() -> (w277:dbl)
        n144 = local read "fft - df"() -> (w274:dbl)
        n145 = local read "fft - f0"() -> (w273:dbl)
        n146 = Bundle("total output power (W)"=w266, "efficiency (%)"=w265) -> (w269:T14)  [unwired: 1 in]
        n147 = Bundle("total output power (W)"=w266, "power loss (W)"=w264) -> (w268:T15)  [unwired: 1 in]
        n148 = Bundle("total output power (W)"=w266, "input power (W)"=w263) -> (w267:T16)  [unwired: 1 in]
        n149 = Bundle By Name("dt"=w277, "Y"=w278) -> (→"Time domain graph":waveform(dbl))  [unwired: 1 in]
        n150 = Bundle("fft - f0"=w273, "fft - df"=w274, "fft - data"=w275) -> (→"Frequency domain graph":T2)  [unwired: 1 in]
        n151 = Build Array(w269, w268, w267) -> (→"Sweep graph":T17)
      }
      frame "Update Sweep Graph Labels" {
        n152 = Unbundle By Name(w283) -> ("Visible Plot Id"=w281:i32)
        n153 = Index Array(array=string[] ["Efficiency (%)", "Power Loss (W)", "Input Power (W)"], index=w281) -> (element=w280:string)
        n154 = property on="Sweep graph" class="XYGraph (strict)"("YScale.NameLbl.Text"=w280) -> ()  [unwired: 2 in, 2 out]
      }
      frame "Exit" {
        # "This case is triggered to close the User Interface from framework"
        n155 = Flush Queue(queue=w290, error in (no error)=w292) -> (queue out=w289:refnum<queue>, error out=w288:errorcluster)  [unwired: 1 out]
        n156 = Release Queue(queue=w289, force destroy? (F)=TRUE, error in (no error)=w288) -> (error out=w287:errorcluster)  [unwired: 2 out]
      }
      frame "Handle Error" {
      }
    }
    n157 = call <vilib>:"Simple Error Handler.vi"("error in (no error)"=w18) -> ()  [unwired: 4 in, 5 out]
  }
